vi "Write video path.vi"(8 "error in (no error)":errorcluster, 9 "Open? (T)":bool=TRUE, 10 "video path":path, 11 "Video File in":refnum<class "Video File.lvclass">) -> (0 "error out":errorcluster, 3 "Video File out":refnum<class "Video File.lvclass">)   [LabVIEW 2018, in "Video File.lvclass"]
uses:
  Video File.lvclass
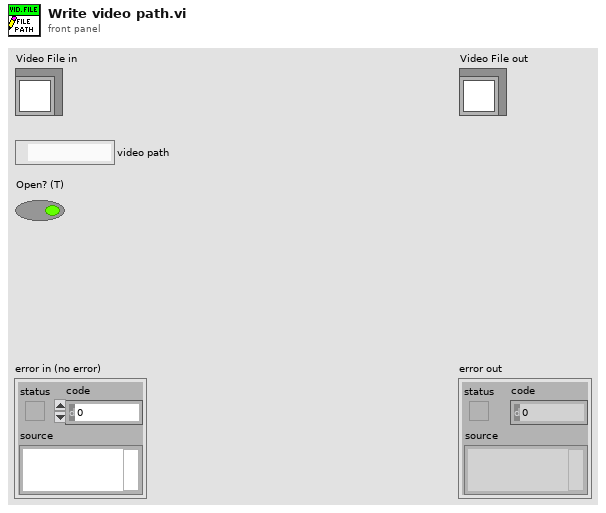
[diagram p1: front panel]
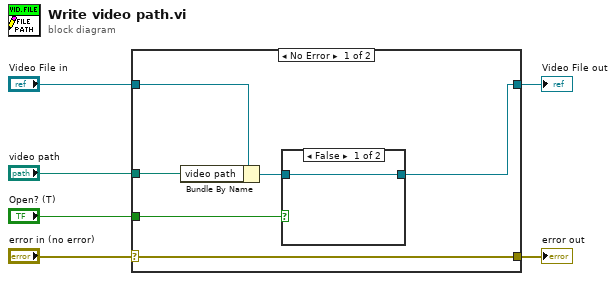
[diagram p0: block diagram]
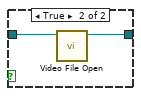
[diagram p2: hidden frame]
diagram:
  n1 = case shown="No Error" "error in (no error)" {
    selector: "error in (no error)" -> [w12 w16]
    tunnel: [w12 w16] -> w5
    tunnel: [w8 w17] -> w3
    tunnel: "Video File in" -> [w11 w17]
    tunnel: "video path" -> [w10 _]
    tunnel: "Open? (T)" -> [w7 _]
    frame No Error {
      n2 = Bundle By Name(cluster=w11, "video path"=w10) -> (w9:refnum<class "Video File.lvclass">)
      n3 = case shown="False" w7 {
        tunnel: w9 -> [w13 w15]
        tunnel: [w13 w14] -> w8
        frame False {
        }
        frame True {
          n4 = call-dynamic "Video File Open.vi"("Video File in"=w15) -> ("Video File out"=w14:refnum<class "Video File.lvclass">)  [unwired: 9 in, 1 out]
        }
      }
    }
    frame Error {
    }
  }
  "error out" <- w5
  "Video File out" <- w3
